vi "run.vi"(8 "error in (no error)":errorcluster, 11 "GeneralAnalyser in":refnum<class "GenericAnalyser.lvclass">) -> (0 "error out":errorcluster, 3 "GeneralAnalyser out":refnum<class "GenericAnalyser.lvclass">)   [LabVIEW 2010, in "GenericAnalyser.lvclass"]
uses:
  GenericAnalyser.lvclass
  common/classes/GenericToplevelComponent/GenericToplevelComponent/common_trigger_enum.ctl
  common/classes/ErrorController/ErrorController/class_data.vi
  common/classes/ErrorController/ErrorController/ErrorController.lvclass
  common/classes/GenericToplevelComponent/GenericToplevelComponent/GenericToplevelComponent.lvclass
panel:
  # "Functionality not available..."
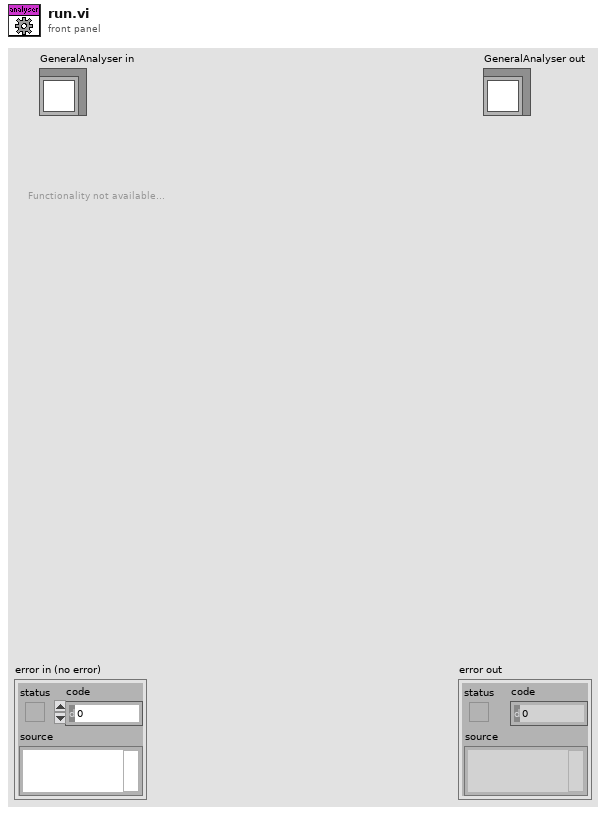
[diagram p1: front panel]
types:
  T1 = typedef "GenericToplevelComponent.lvclass/common_trigger_enum.ctl" = enum16{"NULL", "initialise", "terminate", "fetch command", "fetch data", "attach observer", "register as observer", "detach observer", "acknowledge", "start", "stop", "sweep started", "sweep finished", "experiment started", "experiment stopped"}
  T2 = typedef "main_trigger_enum.ctl" = enum16{"NULL", "initialise", "terminate", "start", "stop", "change objective", "change experimentController", "change imagingMode", "save notebook", "started saving", "finished saving", "expCtr ready", "expCtr missing", "imgMd ready", "imgMd missing", "scanHd ready", "scanHd missing", "DAQ ready", "DAQ missing", "imgAsm ready", "imgAsm missing", "dataColl ready", "dataColl missing", "display ready", "display missing", "analysr ready", "analysr missing", "instrmnt ready", "instrmnt missing", "stimltr ready", "stimltr missing", "stage ready", "stage missing"}
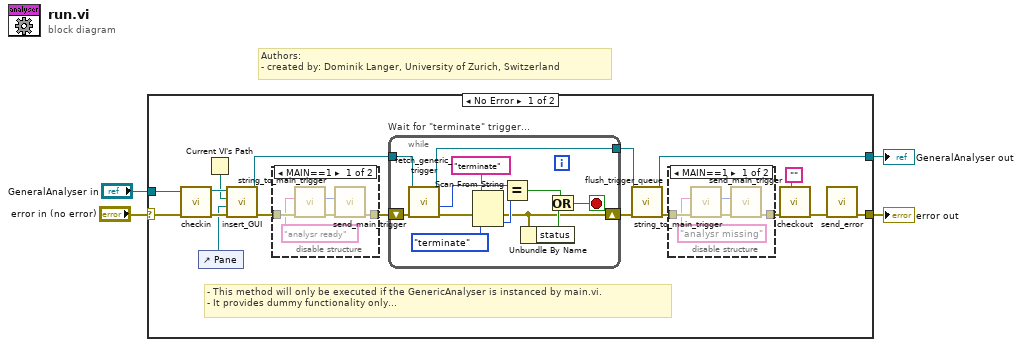
[diagram p0: block diagram]
diagram:
  # "Authors: \n- created by: Dominik Langer, University of Zurich, Switzerland"
  n1 = case shown="No Error" "error in (no error)" {
    selector: "error in (no error)" -> [w21 w47]
    tunnel: [w12 w47] -> w3
    tunnel: [w10 w46] -> w1
    tunnel: "GeneralAnalyser in" -> [w20 w46]
    frame No Error {
      # "- This method will only be executed if the GenericAnalyser is instanced by main.vi.\n- It provides dummy functionality only..."
      n2 = call-dynamic "checkin.vi"("error in (no error)"=w21, "GeneralAnalyser in"=w20) -> ("error out"=w16:errorcluster, "GeneralAnalyser out"=w17:refnum<class "GenericAnalyser.lvclass">)  [unwired: 8 in]
      n3 = control-ref of="Pane"() -> (w14:refnum<vi>)
      n4 = Current VI's Path() -> (path=w15:path)
      n5 = call-dynamic "insert_GUI.vi"("error in (no error)"=w16, "Pane"=w14, "VI path"=w15, "GenericComponent in"=w17) -> ("error out"=w6:errorcluster, "GenericComponent out"=w8:refnum<class "GenericAnalyser.lvclass">)  [unwired: 6 in]
      n6 = disable-structure shown="MAIN==1" {
        disable-tunnel: [w26 w27] -> w5
        disable-tunnel: w6 -> [w25 w27]
        frame condition #0 {
          n7 = call "string_to_main_trigger.vi"("error in (no error)"=w25, "trigger string"="analysr ready") -> ("error out"=w24:errorcluster, "main trigger"=w23:T2)  [unwired: 8 in]
          n8 = call "send_main_trigger.vi"("error in (no error)"=w24, "trigger"=w23) -> ("error out"=w26:errorcluster)  [unwired: 9 in]
        }
        frame condition #1 (active) {
        }
      }
      n9 = while "Wait for \"terminate\" trigger..." {
        tunnel: w8 -> [w42]
        tunnel: [w40] -> w9
        shift-right: [w36] -> w11
        shift-left: w5 -> [w43]
        stop <- w44 stop-if-true
        n10 = call-dynamic "fetch_generic_trigger.vi"("error in (no error)"=w43, "GenericToplevelComponent in"=w42) -> ("error out"=w37:errorcluster, "common trigger"=w35:T1, "GenericToplevelComponent out"=w40:refnum<class "GenericAnalyser.lvclass">)  [unwired: 3 in, 4 out]
        n11 = Scan From String(input string="terminate", error in=w37, default 1=common_trigger_enum."terminate" ("x")) -> (error out=w36:errorcluster, output 1=w38:T1)  [unwired: 2 in, 2 out]
        n12 = Equal?(x=w35, y=w38) -> (x = y?=w41:bool)
        n13 = Unbundle By Name(w36) -> ("status"=w45:bool)
        n14 = Or(x=w41, y=w45) -> (x .or. y?=w44:bool)
      }
      n15 = call-dynamic "flush_trigger_queue.vi"("error in (no error)"=w11, "GenericToplevelComponent in"=w9) -> ("error out"=w7:errorcluster, "GenericToplevelComponent out"=w10:refnum<class "GenericAnalyser.lvclass">)  [unwired: 8 in]
      n16 = disable-structure shown="MAIN==1" {
        disable-tunnel: [w32 w33] -> w18
        disable-tunnel: w7 -> [w31 w33]
        frame condition #0 {
          n17 = call "string_to_main_trigger.vi"("error in (no error)"=w31, "trigger string"="analysr missing") -> ("error out"=w30:errorcluster, "main trigger"=w29:T2)  [unwired: 8 in]
          n18 = call "send_main_trigger.vi"("error in (no error)"=w30, "trigger"=w29) -> ("error out"=w32:errorcluster)  [unwired: 9 in]
        }
        frame condition #1 (active) {
        }
      }
      n19 = call "checkout.vi"("locked by?"="", "error in (no error)"=w18) -> ("error out"=w13:errorcluster)  [unwired: 8 in, 1 out]
      n20 = call "send_error.vi"("error in (no error)"=w13) -> ("error out"=w12:errorcluster)  [unwired: 10 in]
    }
    frame Error {
    }
  }
  "error out" <- w3
  "GeneralAnalyser out" <- w1
